vi "Read SecMirror.lvclass.vi"(8 "error in (no error)":errorcluster, 11 "TelFocus in":refnum<class "TelFocus.lvclass">) -> (0 "error out":errorcluster, 2 "SecMirror.lvclass":refnum<class "SecMirror.lvclass">, 3 "TelFocus out":refnum<class "TelFocus.lvclass">)   [LabVIEW 2018, in "TelFocus.lvclass"]
uses:
  TelFocus.lvclass
  SecMirror/SecMirror.lvclass
  TelFocus.lvclass/TelFocus.ctl
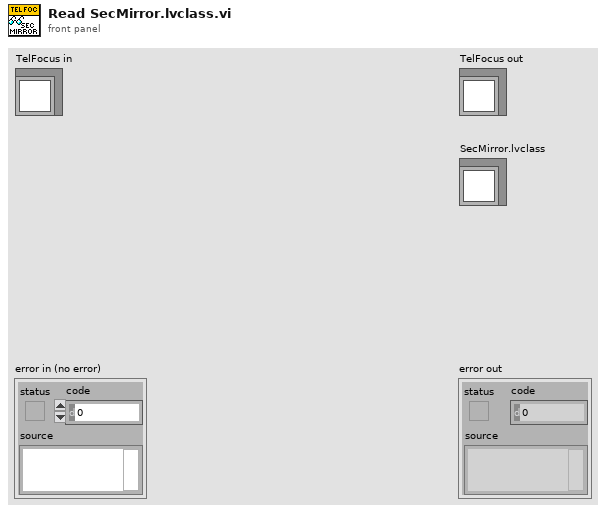
[diagram p1: front panel]
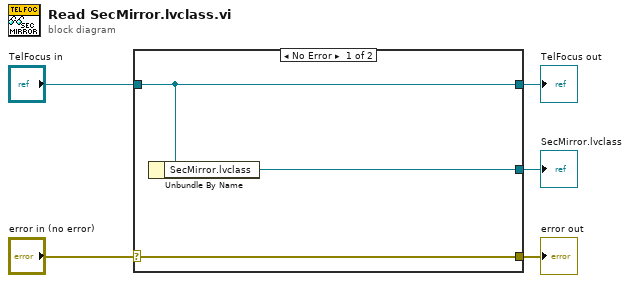
[diagram p0: block diagram]
diagram:
  n1 = case shown="No Error" "error in (no error)" {
    selector: "error in (no error)" -> [w8 w9]
    tunnel: [w8 w9] -> w4
    tunnel: [w7 w10] -> w2
    tunnel: "TelFocus in" -> [w7 w10]
    tunnel: [w6 _] -> w1
    frame No Error {
      n2 = Unbundle By Name(w7) -> ("SecMirror.lvclass"=w6:refnum<class "SecMirror.lvclass">)
    }
    frame Error {
    }
  }
  "error out" <- w4
  "TelFocus out" <- w2
  "SecMirror.lvclass" <- w1
